vi "HasFileBeenModified.vi"(4 "error in (no error)":errorcluster, 7 "Path to Check":path) -> (0 "error out":errorcluster, 1 "FileHasBeenModified?":bool, 2 "FileExists":bool, 3 "dup path":path)   [LabVIEW 2022 SP3]
doc: "Checks if the specified file has been modified since its last recorded modification. Keeps last recorded modification timestamp in memory, and updates this record if the file has been changed since the previous inquiry. To add a file to the tracking list, just specify a unique path that has not been checked since this VI was loaded into memory."
uses:
  ADAM Client/Sub VIs/ADAM Controls/Remember_value_mode.ctl
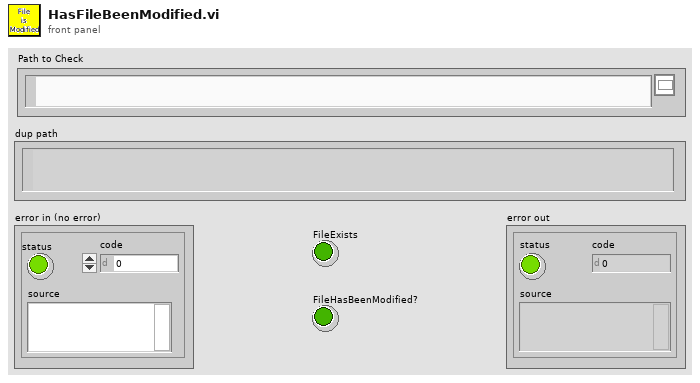
[diagram p1: front panel]
types:
  T1 = typedef "Remember_value_mode.ctl" = enum16{"Read only", "Read and Write"}
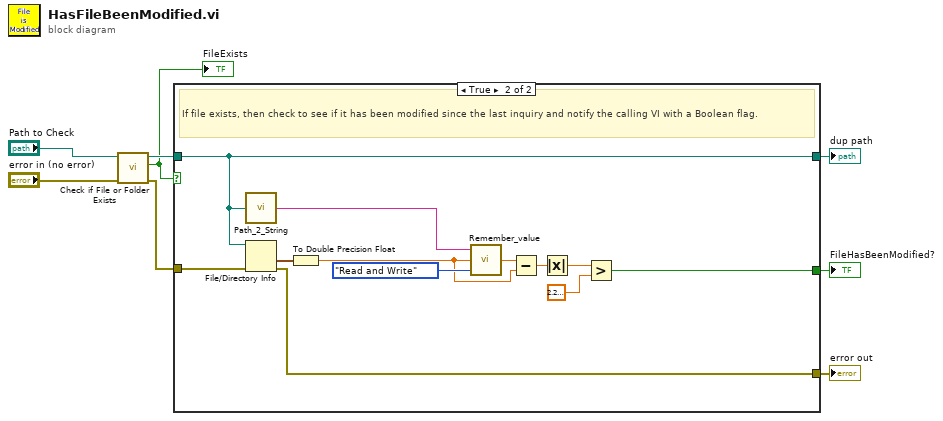
[diagram p0: block diagram]
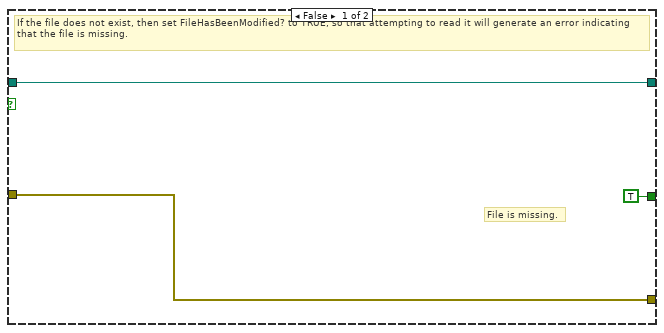
[diagram p2: hidden frame]
diagram:
  n1 = call <vilib>:"Check if File or Folder Exists.vi"("error in (no error)"="error in (no error)", "path"="Path to Check") -> ("error out"=w4:errorcluster, "file or folder exists?"=w1:bool, "dup path"=w7:path)  [unwired: 7 in]
  "FileExists" <- w1
  n2 = case shown="True" w1 {
    tunnel: w7 -> [w11 w22]
    tunnel: [w11 w22] -> w8
    tunnel: [TRUE w14] -> w5
    tunnel: w4 -> [w9 w13]
    tunnel: [w9 w12] -> w2
    frame False {
      # "File is missing."
      # "If the file does not exist, then set FileHasBeenModified? to TRUE, so that attempting to read it will generate an error indicating that the file is missing."
    }
    frame True {
      # "If file exists, then check to see if it has been modified since the last inquiry and notify the calling VI with a Boolean flag."
      n3 = call "Path_2_String.vi"("Real Path"=w22) -> ("Path String"=w20:string)
      n4 = File/Directory Info(path=w22, error in=w13) -> (last mod=w23:timestamp, error out=w12:errorcluster)  [unwired: 5 out]
      n5 = To Double Precision Float(number=w23) -> (double precision float=w18:dbl)
      n6 = call "Remember_value.vi"("Mode"=Remember_value_mode."Read and Write", "Input Value"=w18, "Ch name"=w20) -> ("Output Value"=w19:dbl)
      n7 = Subtract(x=w19, y=w18) -> (x-y=w17:dbl)
      n8 = Absolute Value(x=w17) -> (abs(x)=w16:dbl)
      n9 = Greater?(x=w16, y=2.220446049250313e-16) -> (0:w14:bool)
    }
  }
  "dup path" <- w8
  "FileHasBeenModified?" <- w5
  "error out" <- w2
